vi "Disable_all_channels.vi"(8 "error in":errorcluster, 9 "id_in":i32, 11 "connection ID":refnum<k5>) -> (0 "error out":errorcluster, 1 "id_out":i32, 3 "connection ID out":refnum<k5>)   [LabVIEW 2009]
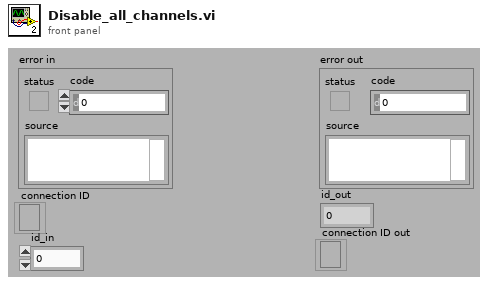
[diagram p1: front panel]
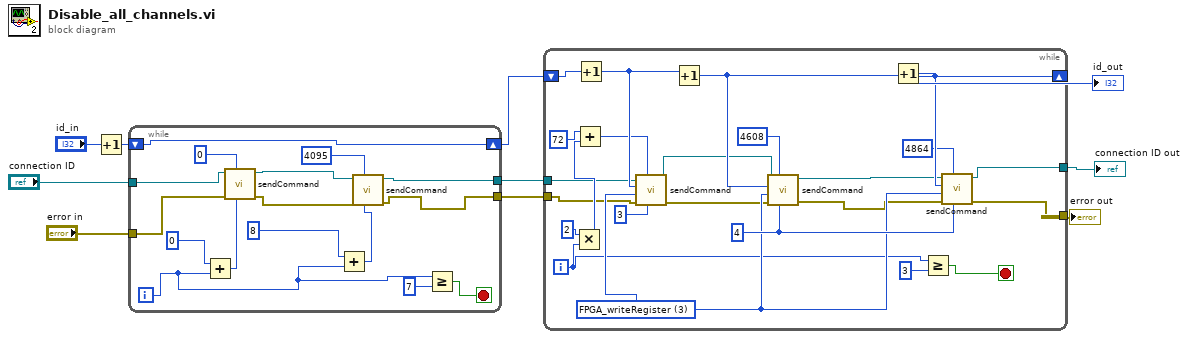
[diagram p0: block diagram]
diagram:
  n1 = Increment(x="id_in") -> (x+1=w3:i32)
  n2 = while {
    tunnel: [w11] -> w6
    tunnel: "error in" -> [w24]
    shift-right: [w19] -> w4
    shift-left: w3 -> [w19]
    tunnel: "connection ID" -> [w15]
    tunnel: [w13] -> w1
    i -> [w17]
    stop <- w18 stop-if-true
    n3 = Add(x=0 ("Address"), y=w17) -> (x+y=w23:i32)
    n4 = call "sendCommand.vi"("Address"=w23, "Data"=0, "error in"=w24, "connection ID"=w15) -> ("error out"=w12:errorcluster, "connection ID out"=w14:refnum<k5>)  [unwired: 3 in, 3 out]
    n5 = Add(x=8 ("Address"), y=w17) -> (x+y=w20:i32)
    n6 = call "sendCommand.vi"("Address"=w20, "Data"=4095, "error in"=w12, "connection ID"=w14) -> ("error out"=w11:errorcluster, "connection ID out"=w13:refnum<k5>)  [unwired: 3 in, 3 out]
    n7 = Greater Or Equal?(x=w17, y=7) -> (x >= y?=w18:bool)
  }
  n8 = while {
    tunnel: [w27] -> w9
    tunnel: [w39] -> w7
    shift-right: [w47] -> w10
    shift-left: w4 -> [w48]
    tunnel: w6 -> [w30]
    tunnel: w1 -> [w31]
    i -> [w34]
    stop <- w32 stop-if-true
    w44 = 4 ("Address")
    w42 = u16 3 items=["sendCommand"=9, "FPGA_writeRegister"=3, "FPGA_readRegister"=2, "uC_writeRegister"=1, "uC_readRegister"=0] ("Action")
    n9 = Multiply(x=2, y=w34) -> (x*y=w37:i32)
    n10 = Add(x=72 ("Data"), y=w37) -> (x+y=w35:i32)
    n11 = Increment(x=w48) -> (x+1=w49:i32)
    n12 = call "sendCommand.vi"("Address"=3, "Data"=w35, "error in"=w30, "Action"=w42, "id_in"=w49, "connection ID"=w31) -> ("error out"=w29:errorcluster, "connection ID out"=w40:refnum<k5>)  [unwired: 1 in, 3 out]
    n13 = Increment(x=w49) -> (x+1=w50:i32)
    n14 = call "sendCommand.vi"("Address"=w44, "Data"=4608, "error in"=w29, "Action"=w42, "id_in"=w50, "connection ID"=w40) -> ("error out"=w28:errorcluster, "connection ID out"=w41:refnum<k5>)  [unwired: 1 in, 3 out]
    n15 = Increment(x=w50) -> (x+1=w47:i32)
    n16 = Greater Or Equal?(x=w34, y=3) -> (x >= y?=w32:bool)
    n17 = call "sendCommand.vi"("Address"=w44, "Data"=4864, "error in"=w28, "Action"=w42, "id_in"=w47, "connection ID"=w41) -> ("error out"=w27:errorcluster, "connection ID out"=w39:refnum<k5>)  [unwired: 1 in, 3 out]
  }
  "error out" <- w9
  "id_out" <- w10
  "connection ID out" <- w7
